vi "Excel - Get Worksheet Reference.vi"(8 "error in (no error)":errorcluster, 11 "Document API in":refnum<class "Document API.lvclass">) -> (0 "error out":errorcluster, 2 "Current Worksheet Reference":refnum<k24>, 3 "Document API out":refnum<class "Document API.lvclass">)   [LabVIEW 2017, in "Document API.lvlib" / "Document API.lvclass"]
uses:
  Document API.lvclass
  C:/Users/Neo/Desktop/Dev_Tools_BR/LabVIEW_NPOI/src/lib/NPOI 2.1.1/NPOI.dll
  lib/NPOI 2.1.1/NPOI.dll
  Document API.lvclass/Document API.ctl
  Get Document Type.vi
  NPOI_Document/npoiDocument/npoiDocument.lvclass
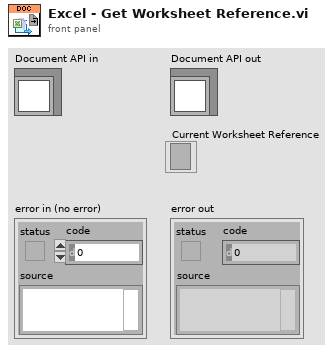
[diagram p1: front panel]
types:
  T1 = typedef "Document API.lvlib/Document API.lvclass/Document Type.ctl" = enum16{"Word", "Excel", "Undefined"}
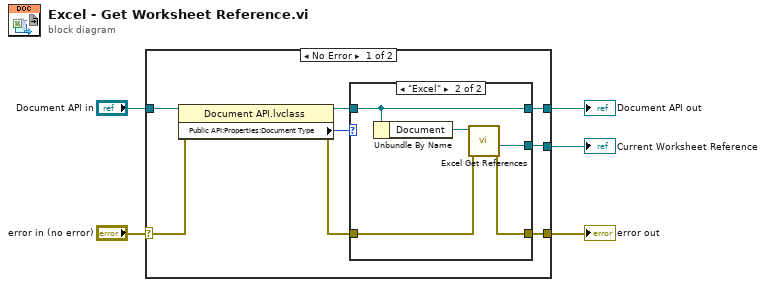
[diagram p0: block diagram]
diagram:
  n1 = case shown="No Error" "error in (no error)" {
    selector: "error in (no error)" -> [w8 w22]
    tunnel: [w12 w22] -> w4
    tunnel: [w10 w21] -> w2
    tunnel: "Document API in" -> [w13 w21]
    tunnel: [w6 _] -> w1
    frame No Error {
      n2 = property class="Document API.lvclass"(reference=w13, error in=w8) -> (reference out=w11:refnum<class "Document API.lvclass">, error out=w7:errorcluster, "Public API:Properties:Document Type"=w9:T1)
      n3 = case shown="\"Excel\"" w9 {
        tunnel: w7 -> [w14 w19]
        tunnel: [w14 w18] -> w12
        tunnel: w11 -> [w15 w17]
        tunnel: [w15 w17] -> w10
        tunnel: [_ w16] -> w6
        frame "Word", Default {
        }
        frame "Excel" {
          n4 = Unbundle By Name(w17) -> ("Document"=w20:refnum<class "npoiDocument.lvclass">)
          n5 = call "Excel Get References.vi"("error in (no error)"=w19, "npoiDocument in"=w20) -> ("error out"=w18:errorcluster, "Current Worksheet.Ref"=w16:refnum<k24>)  [unwired: 6 in, 2 out]
        }
      }
    }
    frame Error {
    }
  }
  "error out" <- w4
  "Document API out" <- w2
  "Current Worksheet Reference" <- w1
